vi "COUNTER_SELECTOR - Type.vi"(8 "error in (no error)":errorcluster) -> (0 "error out":errorcluster, 3 "COUNTER_SELECTOR_VALUE":i32)   [LabVIEW 2015]
doc: "<b>Buffer policy settings can be only unsafe in xiAPI LabVIEW library</b>\nUNSAFE : User gets pointer to internally allocated circle buffer and data may be overwritten by device.\nSAFE : Data from device will be copied to user allocated buffer or xiApi allocated memory."
uses:
  C:/GIT/Cameras3.x/Integrations/Labview/xiLib/xiLIB_32bit/xiLIB/xiCamLib/API/x86/xiApi.NET.dll
  xiLIB_32bit/xiLIB/xiCamLib/API/x86/xiApi.NET.dll
  COUNTER_SELECTOR.ctl
panel:
  in  "COUNTER_SELECTOR":T1
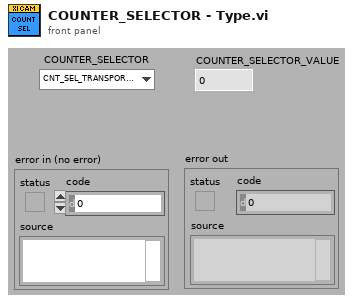
[diagram p1: front panel]
types:
  T1 = typedef "COUNTER_SELECTOR.ctl" = enum16{"CNT_SEL_TRANSPORT_SKIPPED_FRAMES", "CNT_SEL_API_SKIPPED_FRAMES", "CNT_SEL_TRANSPORT_TRANSFERRED_FRAMES"}
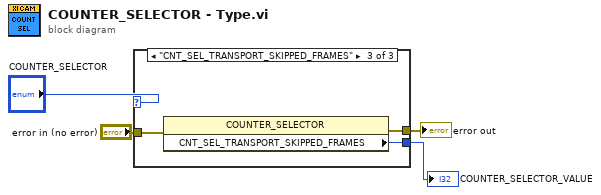
[diagram p0: block diagram]
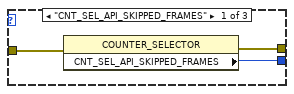
[diagram p2: hidden frame]
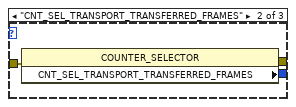
[diagram p3: hidden frame]
diagram:
  n1 = case shown="\"CNT_SEL_TRANSPORT_SKIPPED_FRAMES\"" "COUNTER_SELECTOR" {
    tunnel: "error in (no error)" -> [w7 w10 w13]
    tunnel: [w6 w9 w12] -> w3
    tunnel: [w5 w8 w11] -> w2
    frame "CNT_SEL_API_SKIPPED_FRAMES" {
      n2 = property class="COUNTER_SELECTOR"(error in=w7) -> (error out=w6:errorcluster, "CNT_SEL_API_SKIPPED_FRAMES"=w5:i32)  [unwired: 1 in, 1 out]
    }
    frame "CNT_SEL_TRANSPORT_TRANSFERRED_FRAMES" {
      n3 = property class="COUNTER_SELECTOR"(error in=w10) -> (error out=w9:errorcluster, "CNT_SEL_TRANSPORT_TRANSFERRED_FRAMES"=w8:i32)  [unwired: 1 in, 1 out]
    }
    frame "CNT_SEL_TRANSPORT_SKIPPED_FRAMES" {
      n4 = property class="COUNTER_SELECTOR"(error in=w13) -> (error out=w12:errorcluster, "CNT_SEL_TRANSPORT_SKIPPED_FRAMES"=w11:i32)  [unwired: 1 in, 1 out]
    }
  }
  "error out" <- w3
  "COUNTER_SELECTOR_VALUE" <- w2
